vi "sv_Extract Swept Data to Process.vi"(5 "integration time index in":u32, 6 "waveform data [V]":waveform(dbl)[](array[waveform]), 7 "settle time index in":u32, 8 "error in (no error)":errorcluster, 10 "integration state":bool, 11 "swept sine task in":T1={"source settings"={"AO task name"="", "source"=[]}, "stimulus settings"={"stimulus task name"="", "stimulus"=[]}, "response(s) settings"={"response task name"="", "response"=[]}, "measurement settings"={"AI sampling frequency"=51200.0, "AO sampling frequency"=1024.0, "AI block size"=1024, "AO block Size"=1024, "block duration [ms]"=0.0, "number of AI channels"=0, "device propagation delay [samples]"=0.0, "total propagation time [samples]"=0.0, "DUT propagation time [ms]"=0.0}, "linlog"=enum."linear", "repeat"=enum."off", "frequency list"=[1.0], "amplitude list"=[1.0], "settling time"={"settle time"=0.015599999576807022, "settle cycles"=5}, "integration time"={"integration time"=0.015599999576807022, "integration cycles"=5}, "frequencies indices"={"AI freq index"=0, "AO freq index"=5}, "read marks"={"write index"=0, "read index"=0, "freq start index"=0, "freq stop index"=0, "# extracted"=0, "buffer type"=enum."Invalid buffer", "read/write indices"=[], "AO index"=0, "AI index"=0, "settled"=FALSE, "integration done"=FALSE}, "harmonic settings"={"maximum THD harmonic"=5, "harmonic mapping"=[1], "units"={"THD unit"=enum."%", "nth harmonic unit"=enum."%", "SINAD unit"=enum."dB", "THD+N unit"=enum."dB"}}, "auto resolution settings"={"auto max step"=512, "slow threshold db"=6.0, "fast threshold db"=1.0}, "auto level settings"={"auto level enable"=FALSE, "auto level channel"=6, "ideal ref"=1.0, "max level"=10.0, "ref upper deviation db"=3.0, "ref lower deviation db"=-3.0}, "offset"=1.0, "ramping rate"=0.0, "phase"=1.0, "initialize"=FALSE} {"phase" format="%.2f"; "response(s) settings"."response"."channel info"."pregain" format="%.2f"; "response(s) settings"."response"."channel info"."weighting filter" items=["Linear", "A-weighting", "B-weighting", "C-weighting", "ITU-R 468-4", "Dolby", "CCITT", "C-message", "Wb", "Wc", "Wd", "We", "Wf", "Wh", "Wj", "Wk", "Wm", "AES17 20 kHz lowpass", "AES17 40 kHz lowpass", "AES17 20 kHz highpass", "AES17 40 kHz highpass"]; "response(s) settings"."response"."channel info"."dB reference" format="%^.1e"; "response(s) settings"."response"."channel info"."engineering units" items=["custom..."=0, "V"=1, "A"=21, "C"=30, "pC"=31, "s"=32, "-"=29, "Pa"=2, "N"=20, "g"=3, "m/s^2"=4, "m/s"=5, "m"=6, "mm/s"=12, "mm"=13, "micron/s"=14, "micron"=15, "in/s^2"=7, "in/s"=8, "in"=9, "mil/s"=10, "mil"=11, "rad/s^2"=16, "rad/s"=17, "rad"=18, "deg/s^2"=26, "deg/s"=27, "deg"=28, "RPM"=22, "cycle/s^2"=23, "Hz"=24, "cycle"=25, "strain"=19]; "response(s) settings"."response"."channel info"."sensor sensitivity" format="%#_5f"; "stimulus settings"."stimulus"."channel info"."pregain" format="%.2f"; "stimulus settings"."stimulus"."channel info"."weighting filter" items=["Linear", "A-weighting", "B-weighting", "C-weighting", "ITU-R 468-4", "Dolby", "CCITT", "C-message", "Wb", "Wc", "Wd", "We", "Wf", "Wh", "Wj", "Wk", "Wm", "AES17 20 kHz lowpass", "AES17 40 kHz lowpass", "AES17 20 kHz highpass", "AES17 40 kHz highpass"]; "stimulus settings"."stimulus"."channel info"."dB reference" format="%^.1e"; "stimulus settings"."stimulus"."channel info"."engineering units" items=["custom..."=0, "V"=1, "A"=21, "C"=30, "pC"=31, "s"=32, "-"=29, "Pa"=2, "N"=20, "g"=3, "m/s^2"=4, "m/s"=5, "m"=6, "mm/s"=12, "mm"=13, "micron/s"=14, "micron"=15, "in/s^2"=7, "in/s"=8, "in"=9, "mil/s"=10, "mil"=11, "rad/s^2"=16, "rad/s"=17, "rad"=18, "deg/s^2"=26, "deg/s"=27, "deg"=28, "RPM"=22, "cycle/s^2"=23, "Hz"=24, "cycle"=25, "strain"=19]; "stimulus settings"."stimulus"."channel info"."sensor sensitivity" format="%#_5f"; "ramping rate" format="%.4f"; "offset" format="%.2f"; "auto level settings"."ref lower deviation db" format="%.4f"; "auto level settings"."ref upper deviation db" format="%.4f"; "auto level settings"."max level" format="%.4f"; "auto level settings"."ideal ref" format="%.4f"; "auto resolution settings"."fast threshold db" format="%.4f"; "auto resolution settings"."slow threshold db" format="%.4f"; "harmonic settings"."maximum THD harmonic" max=10 step=1; "integration time"."integration time" format="%.2p"; "settling time"."settle time" format="%.2p"; "amplitude list" format="%.2f"; "frequency list" format="%.2f"; "measurement settings"."DUT propagation time [ms]" format="%.2f"; "measurement settings"."AO sampling frequency" format="%.2f"; "measurement settings"."AI sampling frequency" format="%.2f"}) -> (0 "error out":errorcluster, 3 "swept sine task out":T1={"source settings"={"AO task name"="", "source"=[]}, "stimulus settings"={"stimulus task name"="", "stimulus"=[]}, "response(s) settings"={"response task name"="", "response"=[]}, "measurement settings"={"AI sampling frequency"=51200.0, "AO sampling frequency"=1024.0, "AI block size"=1024, "AO block Size"=1024, "block duration [ms]"=0.0, "number of AI channels"=0, "device propagation delay [samples]"=0.0, "total propagation time [samples]"=0.0, "DUT propagation time [ms]"=0.0}, "linlog"=enum."linear", "repeat"=enum."off", "frequency list"=[1.0], "amplitude list"=[1.0], "settling time"={"settle time"=0.015599999576807022, "settle cycles"=5}, "integration time"={"integration time"=0.015599999576807022, "integration cycles"=5}, "frequencies indices"={"AI freq index"=0, "AO freq index"=5}, "read marks"={"write index"=0, "read index"=0, "freq start index"=0, "freq stop index"=0, "# extracted"=0, "buffer type"=enum."Invalid buffer", "read/write indices"=[], "AO index"=0, "AI index"=0, "settled"=FALSE, "integration done"=FALSE}, "harmonic settings"={"maximum THD harmonic"=5, "harmonic mapping"=[1], "units"={"THD unit"=enum."%", "nth harmonic unit"=enum."%", "SINAD unit"=enum."dB", "THD+N unit"=enum."dB"}}, "auto resolution settings"={"auto max step"=512, "slow threshold db"=6.0, "fast threshold db"=1.0}, "auto level settings"={"auto level enable"=FALSE, "auto level channel"=6, "ideal ref"=1.0, "max level"=10.0, "ref upper deviation db"=3.0, "ref lower deviation db"=-3.0}, "offset"=1.0, "ramping rate"=0.0, "phase"=1.0, "initialize"=FALSE} {"phase" format="%.2f"; "response(s) settings"."response"."channel info"."pregain" format="%.2f"; "response(s) settings"."response"."channel info"."weighting filter" items=["Linear", "A-weighting", "B-weighting", "C-weighting", "ITU-R 468-4", "Dolby", "CCITT", "C-message", "Wb", "Wc", "Wd", "We", "Wf", "Wh", "Wj", "Wk", "Wm", "AES17 20 kHz lowpass", "AES17 40 kHz lowpass", "AES17 20 kHz highpass", "AES17 40 kHz highpass"]; "response(s) settings"."response"."channel info"."dB reference" format="%^.1e"; "response(s) settings"."response"."channel info"."engineering units" items=["custom..."=0, "V"=1, "A"=21, "C"=30, "pC"=31, "s"=32, "-"=29, "Pa"=2, "N"=20, "g"=3, "m/s^2"=4, "m/s"=5, "m"=6, "mm/s"=12, "mm"=13, "micron/s"=14, "micron"=15, "in/s^2"=7, "in/s"=8, "in"=9, "mil/s"=10, "mil"=11, "rad/s^2"=16, "rad/s"=17, "rad"=18, "deg/s^2"=26, "deg/s"=27, "deg"=28, "RPM"=22, "cycle/s^2"=23, "Hz"=24, "cycle"=25, "strain"=19]; "response(s) settings"."response"."channel info"."sensor sensitivity" format="%#_5f"; "stimulus settings"."stimulus"."channel info"."pregain" format="%.2f"; "stimulus settings"."stimulus"."channel info"."weighting filter" items=["Linear", "A-weighting", "B-weighting", "C-weighting", "ITU-R 468-4", "Dolby", "CCITT", "C-message", "Wb", "Wc", "Wd", "We", "Wf", "Wh", "Wj", "Wk", "Wm", "AES17 20 kHz lowpass", "AES17 40 kHz lowpass", "AES17 20 kHz highpass", "AES17 40 kHz highpass"]; "stimulus settings"."stimulus"."channel info"."dB reference" format="%^.1e"; "stimulus settings"."stimulus"."channel info"."engineering units" items=["custom..."=0, "V"=1, "A"=21, "C"=30, "pC"=31, "s"=32, "-"=29, "Pa"=2, "N"=20, "g"=3, "m/s^2"=4, "m/s"=5, "m"=6, "mm/s"=12, "mm"=13, "micron/s"=14, "micron"=15, "in/s^2"=7, "in/s"=8, "in"=9, "mil/s"=10, "mil"=11, "rad/s^2"=16, "rad/s"=17, "rad"=18, "deg/s^2"=26, "deg/s"=27, "deg"=28, "RPM"=22, "cycle/s^2"=23, "Hz"=24, "cycle"=25, "strain"=19]; "stimulus settings"."stimulus"."channel info"."sensor sensitivity" format="%#_5f"; "ramping rate" format="%.4f"; "offset" format="%.2f"; "auto level settings"."ref lower deviation db" format="%.4f"; "auto level settings"."ref upper deviation db" format="%.4f"; "auto level settings"."max level" format="%.4f"; "auto level settings"."ideal ref" format="%.4f"; "auto resolution settings"."fast threshold db" format="%.4f"; "auto resolution settings"."slow threshold db" format="%.4f"; "harmonic settings"."maximum THD harmonic" max=10 step=1; "integration time"."integration time" format="%.2p"; "settling time"."settle time" format="%.2p"; "amplitude list" format="%.2f"; "frequency list" format="%.2f"; "measurement settings"."DUT propagation time [ms]" format="%.2f"; "measurement settings"."AO sampling frequency" format="%.2f"; "measurement settings"."AI sampling frequency" format="%.2f"}, 4 "data to process [V]":cluster{"stimulus":dbl[], "response":dbl[]} {"response" format="%.2f"; "stimulus" format="%.2f"})   [LabVIEW 2017, in "SoundVib_SweptSine.lvlib"]
uses:
  <vilib>/addons/Sound and Vibration/svt_Swept Sine/SoundVib_SweptSine.lvlib
  <vilib>/addons/Sound and Vibration/svt_Swept Sine/subVIs/sv_Swept Sine Task.ctl
  <vilib>/addons/_NISVFA/_Shared subVIs/Controls/svc_Channel Info.ctl
  <vilib>/addons/_NISVFA/_Shared subVIs/Controls/svc_Engineering Units Text Ring.ctl
  <vilib>/addons/_NISVFA/_Shared subVIs/Controls/svc_Weighting Filter Text Ring.ctl
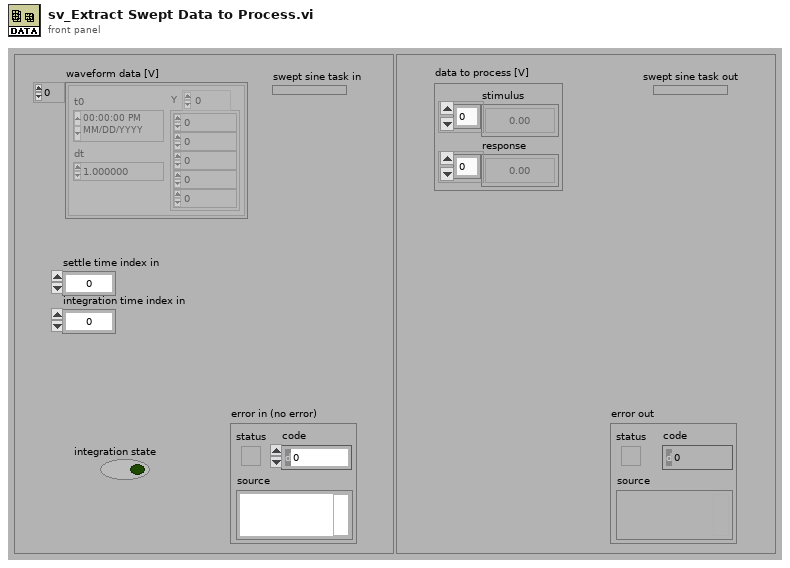
[diagram p1: front panel]
types:
  T1 = typedef "SoundVib_SweptSine.lvlib/sv_Swept Sine Task.ctl" = cluster{"source settings":cluster{"AO task name":refnum<k21>, "source":cluster{"AO physical channel":tag}[]}, "stimulus settings":cluster{"stimulus task name":refnum<k21>, "stimulus":cluster{"stimulus physical channel":tag, "channel info":T2}[]}, "response(s) settings":cluster{"response task name":refnum<k21>, "response":cluster{"response physical channel":tag, "channel info":T2}[]}, "measurement settings":cluster{"AI sampling frequency":dbl, "AO sampling frequency":dbl, "AI block size":i32, "AO block Size":i32, "block duration [ms]":dbl, "number of AI channels":i32, "device propagation delay [samples]":dbl, "total propagation time [samples]":dbl, "DUT propagation time [ms]":dbl}, "linlog":enum16{"linear", "log"}, "repeat":enum16{"off", "on"}, "frequency list":dbl[], "amplitude list":dbl[], "settling time":cluster{"settle time":dbl, "settle cycles":i32}, "integration time":cluster{"integration time":dbl, "integration cycles":i32}, "frequencies indices":cluster{"AI freq index":i32, "AO freq index":i32}, "read marks":cluster{"write index":u32, "read index":u32, "freq start index":u32, "freq stop index":u32, "# extracted":u32, "buffer type":enum16{"Invalid buffer", "Intermediate buffer", "Final buffer"}, "read/write indices":cluster{"settle time index":u32, "integration time index":u32}[], "AO index":i32, "AI index":i32, "settled":bool, "integration done":bool}, "harmonic settings":cluster{"maximum THD harmonic":u32, "harmonic mapping":u32[], "units":cluster{"THD unit":enum16{"dB", "%"}, "nth harmonic unit":enum16{"dB", "%"}, "SINAD unit":enum16{"dB", "%"}, "THD+N unit":enum16{"dB", "%"}}}, "auto resolution settings":cluster{"auto max step":i32, "slow threshold db":dbl, "fast threshold db":dbl}, "auto level settings":cluster{"auto level enable":bool, "auto level channel":u8, "ideal ref":sgl, "max level":sgl, "ref upper deviation db":sgl, "ref lower deviation db":sgl}, "offset":dbl, "ramping rate":dbl, "phase":dbl, "initialize":bool}
  T2 = typedef "svc_Channel Info.ctl" = cluster{"sensor sensitivity":dbl, "engineering units":T3, "dB reference":dbl, "custom label":string, "weighting filter":T4, "pregain":dbl}
  T3 = typedef "svc_Engineering Units Text Ring.ctl" = u16
  T4 = typedef "svc_Weighting Filter Text Ring.ctl" = u16
  T5 = enum16{"Invalid buffer", "Intermediate buffer", "Final buffer"}
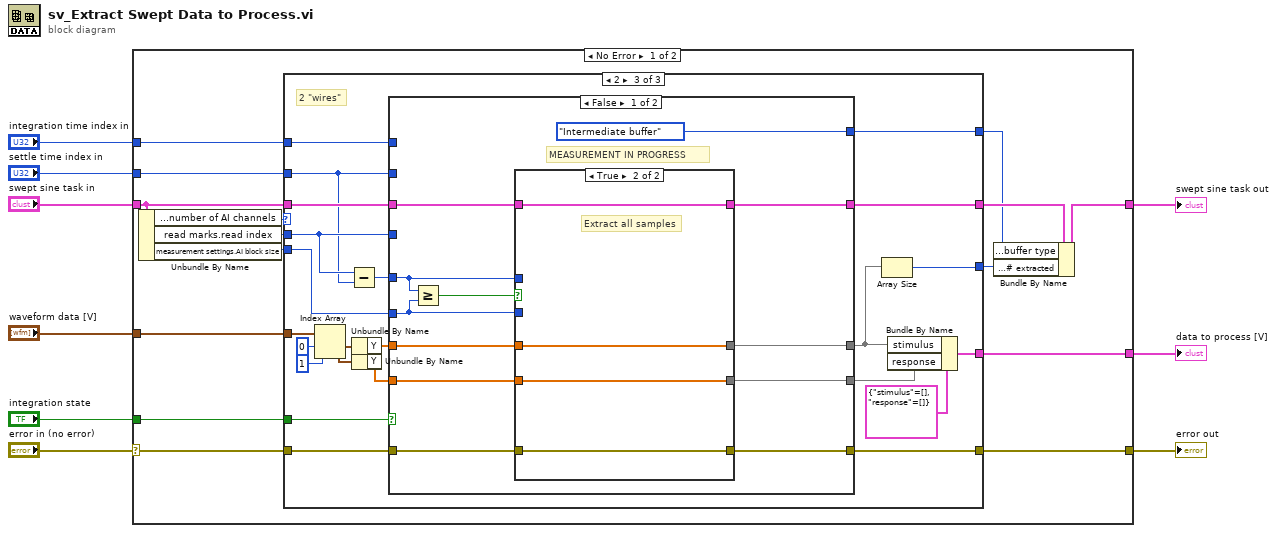
[diagram p0: block diagram]
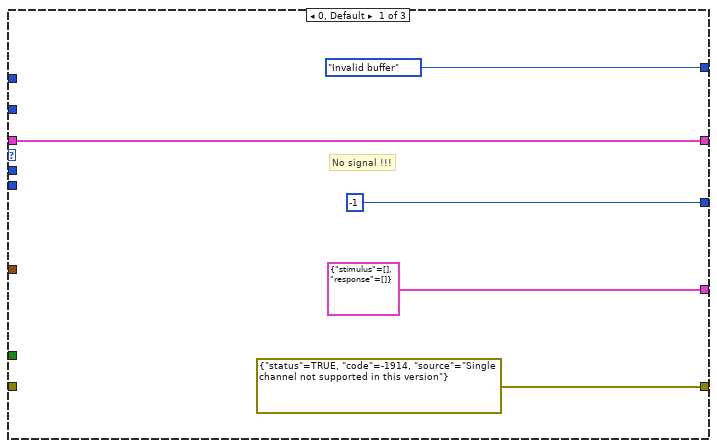
[diagram p2: hidden frame]
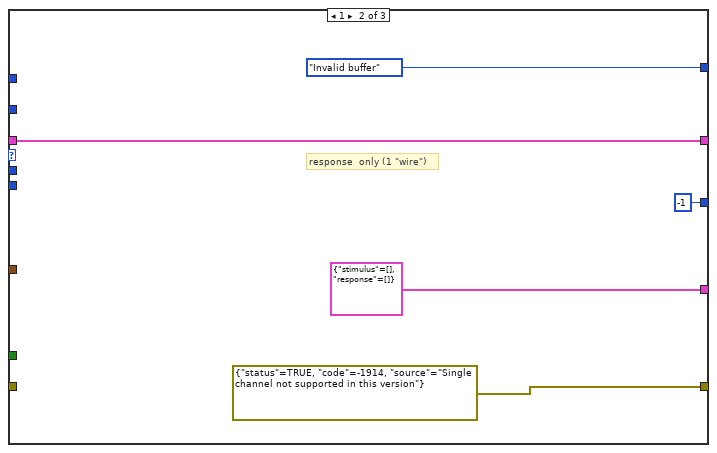
[diagram p3: hidden frame]
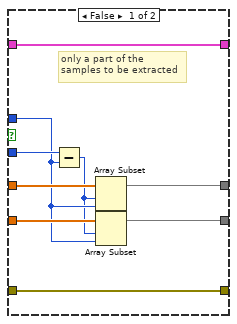
[diagram p4: hidden frame]
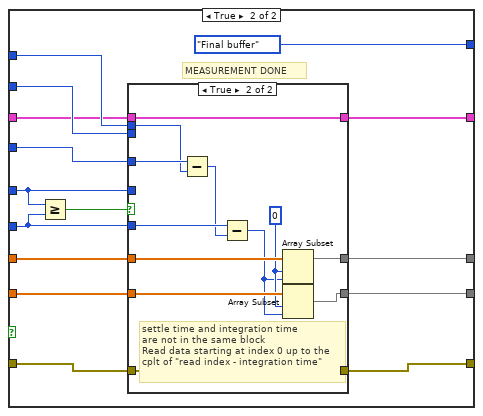
[diagram p5: hidden frame]
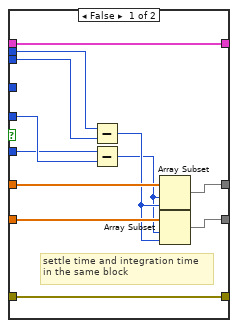
[diagram p6: hidden frame]
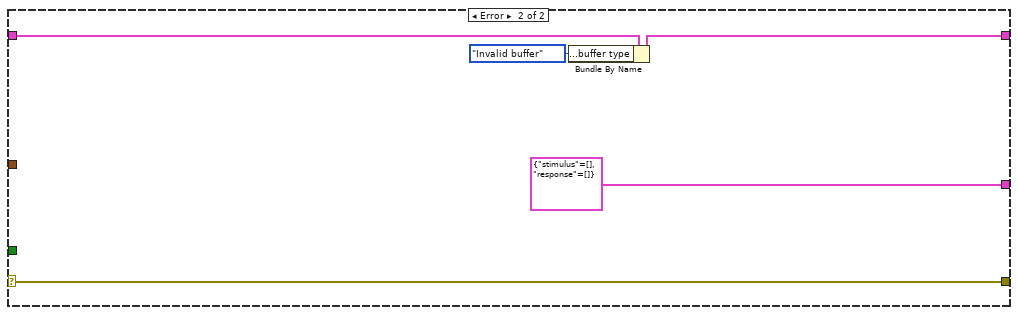
[diagram p7: hidden frame]
diagram:
  n1 = case shown="No Error" "error in (no error)" {
    selector: "error in (no error)" -> [w22 w126]
    tunnel: "swept sine task in" -> [w19 w123]
    tunnel: [w16 w122] -> w4
    tunnel: "waveform data [V]" -> [w23 _]
    tunnel: [w21 w126] -> w6
    tunnel: [w24 cluster{"stimulus":dbl[], "response":dbl[]} {"stimulus"=[], "response"=[]} ("data to process")] -> w5
    tunnel: "integration state" -> [w20 _]
    tunnel: "settle time index in" -> [w13 _]
    tunnel: "integration time index in" -> [w12 _]
    frame No Error {
      n2 = Unbundle By Name(w19) -> ("measurement settings.number of AI channels"=w18:i32, "read marks.read index"=w10:u32, "measurement settings.AI block size"=w11:i32)
      n3 = case shown="2" w18 {
        tunnel: [cluster{"stimulus":dbl[], "response":dbl[]} {"stimulus"=[], "response"=[]} ("data to process") cluster{"stimulus":dbl[], "response":dbl[]} {"stimulus"=[], "response"=[]} ("data to process") w52] -> w24
        tunnel: w19 -> [w29 w34 w37]
        tunnel: [w29 w34 w43] -> w17
        tunnel: w23 -> [_ _ w44]
        tunnel: w22 -> [_ _ w47]
        tunnel: [errorcluster {"status"=TRUE, "code"=-1914, "source"="Single channel not supported in this version"} ("error IO") errorcluster {"status"=TRUE, "code"=-1914, "source"="Single channel not supported in this version"} ("error IO") w46] -> w21
        tunnel: w20 -> [_ _ w45]
        tunnel: [-1 -1 w42] -> w15
        tunnel: [T5."Invalid buffer" ("buffer type") T5."Invalid buffer" ("buffer type") w41] -> w14
        tunnel: w13 -> [_ _ w35]
        tunnel: w12 -> [_ _ w36]
        tunnel: w11 -> [_ _ w39]
        tunnel: w10 -> [_ _ w38]
        frame 0, Default {
          # "No signal !!!"
        }
        frame 1 {
          # "response  only (1 \"wire\")"
        }
        frame 2 {
          # "2 \"wires\""
          n4 = Index Array(array=w44, index #1=0 ("index"), index #2=1 ("index")) -> (element #1=w57:waveform(dbl), element #2=w54:waveform(dbl))
          n5 = Subtract(x=w38, y=w35) -> (x-y=w40:u32)
          n6 = Unbundle By Name(w57) -> ("Y"=w51:dbl[])
          n7 = Unbundle By Name(w54) -> ("Y"=w50:dbl[])
          n8 = case shown="False" w45 {
            tunnel: w37 -> [w58 w84]
            tunnel: w51 -> [w68 w97]
            tunnel: w50 -> [w66 w95]
            tunnel: [w67 w96] -> w48
            tunnel: [w65 w94] -> w49
            tunnel: [w64 w93] -> w43
            tunnel: w47 -> [w63 w91]
            tunnel: [w62 w90] -> w46
            tunnel: [T5."Intermediate buffer" ("buffer type") T5."Final buffer" ("buffer type")] -> w41
            tunnel: w39 -> [w60 w83]
            tunnel: w40 -> [w59 w88]
            tunnel: w38 -> [_ w87]
            tunnel: w35 -> [_ w86]
            tunnel: w36 -> [_ w85]
            frame False {
              # "MEASUREMENT IN PROGRESS"
              n9 = Greater Or Equal?(x=w59, y=w60) -> (x >= y?=w69:bool)
              n10 = case shown="True" w69 {
                tunnel: w68 -> [w78 w82]
                tunnel: [w77 w82] -> w67
                tunnel: w66 -> [w76 w81]
                tunnel: [w75 w81] -> w65
                tunnel: w60 -> [w74 _]
                tunnel: w59 -> [w71 _]
                tunnel: w58 -> [w73 w80]
                tunnel: [w73 w80] -> w64
                tunnel: w63 -> [w72 w79]
                tunnel: [w72 w79] -> w62
                frame False {
                  # "only a part of the \nsamples to be extracted"
                  n11 = Subtract(x=w74, y=w71) -> (x-y=w70:u32)
                  n12 = Array Subset(array=w78, index=w70, length=w71) -> (w77:dbl[])
                  n13 = Array Subset(array=w76, index=w70, length=w71) -> (w75:dbl[])
                }
                frame True {
                  # "Extract all samples"
                }
              }
            }
            frame True {
              # "MEASUREMENT DONE"
              n14 = Greater Or Equal?(x=w88, y=w83) -> (x >= y?=w89:bool)
              n15 = case shown="True" w89 {
                tunnel: w87 -> [_ w114]
                tunnel: w97 -> [w109 w121]
                tunnel: w85 -> [w105 w113]
                tunnel: [w106 w120] -> w96
                tunnel: w95 -> [w108 w119]
                tunnel: [w107 w118] -> w94
                tunnel: w83 -> [w98 w112]
                tunnel: w86 -> [w103 _]
                tunnel: w84 -> [w102 w117]
                tunnel: [w102 w117] -> w93
                tunnel: w91 -> [w101 w116]
                tunnel: [w101 w116] -> w90
                tunnel: w88 -> [w99 _]
                frame False {
                  # "settle time and integration time \nin the same block"
                  n16 = Subtract(x=w105, y=w103) -> (x-y=w104:u32)
                  n17 = Subtract(x=w98, y=w99) -> (x-y=w100:u32)
                  n18 = Array Subset(array=w109, index=w100, length=w104) -> (w106:dbl[])
                  n19 = Array Subset(array=w108, index=w100, length=w104) -> (w107:dbl[])
                }
                frame True {
                  w115 = 0 ("index")
                  # "settle time and integration time \nare not in the same block\nRead data starting at index 0 up to the \ncplt of \"read index - integration time\""
                  n20 = Subtract(x=w114, y=w113) -> (x-y=w111:u32)
                  n21 = Subtract(x=w112, y=w111) -> (x-y=w110:u32)
                  n22 = Array Subset(array=w121, index=w115, length=w110) -> (w120:dbl[])
                  n23 = Array Subset(array=w119, index=w115, length=w110) -> (w118:dbl[])
                }
              }
            }
          }
          n24 = Array Size(array=w48) -> (size(s)=w42:i32)
          n25 = Bundle By Name(cluster=cluster{"stimulus":dbl[], "response":dbl[]} {"stimulus"=[], "response"=[]} ("data to process"), "stimulus"=w48, "response"=w49) -> (w52:cluster{"stimulus":dbl[], "response":dbl[]})
        }
      }
      n26 = Bundle By Name(cluster=w17, "read marks.buffer type"=w14, "read marks.# extracted"=w15) -> (w16:T1)
    }
    frame Error {
      n27 = Bundle By Name(cluster=w123, "read marks.buffer type"=T5."Invalid buffer" ("buffer type")) -> (w122:T1)
    }
  }
  "error out" <- w6
  "swept sine task out" <- w4
  "data to process [V]" <- w5
